vi "RudderForceBalanceTest-OLD.vi"() -> (3 "Were there any errors at all?":bool)   [LabVIEW 2013]
panel:
  out "Are Jib Suggestions Right?":bool[](array[boolean])
  out "Are Main Suggestion Right?":bool[](array[boolean])
  out "Actual Jib Sail Suggestions":dbl[](array[numeric])
  out "Actual Main Sail Suggestions":dbl[](array[numeric])
  in  "Expected Jib Outputs":dbl[](array[numeric])=[0.0, 0.0]
  in  "Expected Main Outputs":dbl[](array[numeric])=[0.0, 0.0]
  in  "Inputs":dbl[](array[numeric])=[0.0, 1.0]
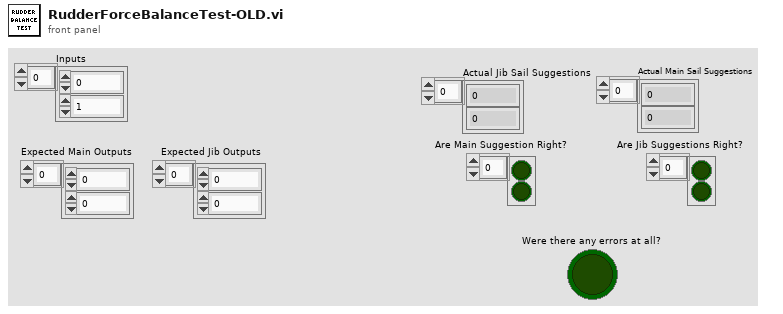
[diagram p1: front panel]
types:
  T1 = typedef "Sail Set Suggestions.ctl" = cluster{"MainSailSuggestion":dbl, "JibSailSuggestion":dbl}
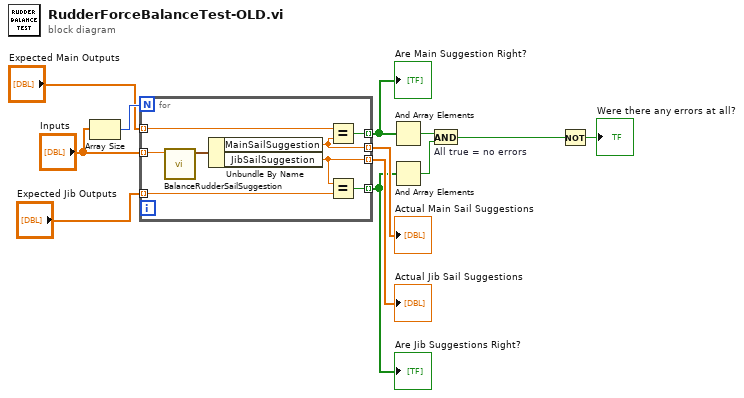
[diagram p0: block diagram]
diagram:
  n1 = Array Size(array="Inputs") -> (size(s)=w12:i32)
  n2 = for {
    N: w12 -> [_]
    tunnel: "Inputs" -> [w16] mode=indexing
    tunnel: "Expected Main Outputs" -> [w20] mode=indexing
    tunnel: "Expected Jib Outputs" -> [w14] mode=indexing
    tunnel: [w19] -> w8 mode=indexing
    tunnel: [w13] -> w7 mode=indexing
    tunnel: [w18] -> w4 mode=indexing
    tunnel: [w17] -> w6 mode=indexing
    n3 = call "BalanceRudderSailSuggestion.vi"("ForceOnRudder"=w16) -> ("Suggested Sail Setpoints"=w15:T1)  [unwired: 10 in]
    n4 = Unbundle By Name(w15) -> ("MainSailSuggestion"=w19:dbl, "JibSailSuggestion"=w13:dbl)
    n5 = Equal?(x=w20, y=w19) -> (x = y?=w18:bool)
    n6 = Equal?(x=w13, y=w14) -> (x = y?=w17:bool)
  }
  "Actual Main Sail Suggestions" <- w8
  "Actual Jib Sail Suggestions" <- w7
  "Are Main Suggestion Right?" <- w4
  "Are Jib Suggestions Right?" <- w6
  n7 = And Array Elements(Boolean array=w4) -> (logical AND=w3:bool)
  n8 = And Array Elements(Boolean array=w6) -> (logical AND=w5:bool)
  n9 = And "All true = no errors"(x=w3, y=w5) -> (x .and. y?=w2:bool)
  n10 = Not(x=w2) -> (.not. x?=→"Were there any errors at all?":bool)
